vi "Replace Control.vi"(6 "Palette String":string, 8 "error in (no error)":errorcluster, 9 "Path":path, 11 "Ctl Refnum":refnum<vi>) -> (0 "error out":errorcluster, 3 "New Node Refnum":refnum<vi>)   [LabVIEW 2018, in "Scripting Tools.lvlib"]
uses:
  Scripting Tools.lvlib
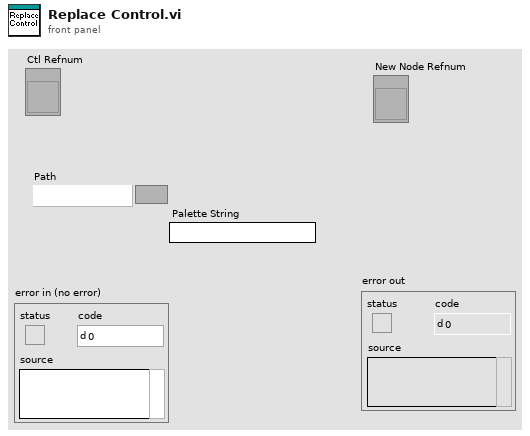
[diagram p1: front panel]
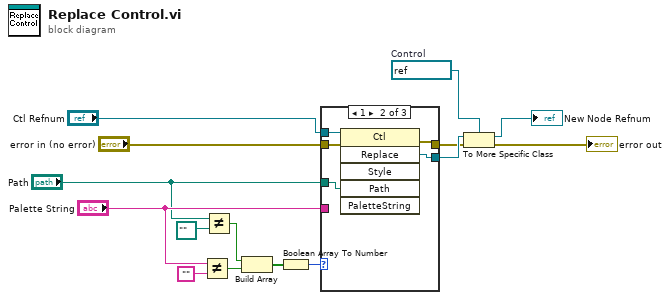
[diagram p0: block diagram]
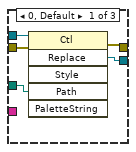
[diagram p2: hidden frame]
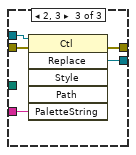
[diagram p3: hidden frame]
diagram:
  w8 = refnum<vi> refnum  # Control
  n1 = Not Equal?(x="Palette String", y="") -> (x != y?=w11:bool)
  n2 = Not Equal?(x="Path", y=path "") -> (x != y?=w12:bool)
  n3 = Build Array(w12, w11) -> (w10:bool[])
  n4 = Boolean Array To Number(Boolean array=w10) -> (number=w7:u32)
  n5 = case shown="1" w7 {
    tunnel: "Ctl Refnum" -> [w20 w25 w30]
    tunnel: [w19 w24 w29] -> w9
    tunnel: "Palette String" -> [_ _ w28]
    tunnel: "Path" -> [w18 w23 _]
    tunnel: "error in (no error)" -> [w17 w22 w27]
    tunnel: [w16 w21 w26] -> w2
    frame 0, Default {
      n6 = invoke class="Ctl" method="Replace"(reference=w20, error in=w17, "Path"=w18) -> (error out=w16:errorcluster, "Replace"=w19:refnum<vi>)  [unwired: 3 in, 4 out]
    }
    frame 1 {
      n7 = invoke class="Ctl" method="Replace"(reference=w25, error in=w22, "Path"=w23) -> (error out=w21:errorcluster, "Replace"=w24:refnum<vi>)  [unwired: 3 in, 4 out]
    }
    frame 2, 3 {
      n8 = invoke class="Ctl" method="Replace"(reference=w30, error in=w27, "PaletteString"=w28) -> (error out=w26:errorcluster, "Replace"=w29:refnum<vi>)  [unwired: 3 in, 4 out]
    }
  }
  n9 = To More Specific Class(target class=w8, reference=w9, error in=w2) -> (specific class reference=→"New Node Refnum":refnum<vi>, error out=→"error out":errorcluster)
